vi "Create Plot Object.vi"(6 "Control Ref Queue":T1, 7 "Actual Transform In":T2, 8 "error in (no error)":errorcluster, 9 "Multiplot Representation In":T4, 10 "3D Stem.lvclass in":refnum<class "3D Stem.lvclass">, 11 "Plot Object In":refnum<vi>) -> (0 "error out":errorcluster, 1 "Multiplot Representation Out":T4, 2 "3D Stem.lvclass out":refnum<class "3D Stem.lvclass">, 3 "Plot Object Out":refnum<vi>, 5 "Actual Transform Out":T2)   [LabVIEW 2020, in "3D Stem.lvclass"]
uses:
  <vilib>/Math Plots/3D Math Plots/3D Stem/3D Stem/3D Stem.lvclass
  <vilib>/Math Plots/3D Math Plots/3D Plot/3D Plot/Typedef/Multiplot Representation.ctl
  <vilib>/Math Plots/3D Math Plots/3D Plot/3D Plot/Typedef/Plot Representation.ctl
  <vilib>/Math Plots/3D Math Plots/3D Plot/3D Plot/Typedef/Range Clusters.ctl
  <vilib>/Math Plots/3D Math Plots/3D Plot/3D Plot/Typedef/Mesh Data.ctl
  <vilib>/Math Plots/3D Math Plots/3D Plot/3D Plot/Typedef/Actual Transform.ctl
  <vilib>/Math Plots/3D Math Plots/3D Plot/Action String/3DMathPlot Ctrl Act Queue.ctl
  <vilib>/Math Plots/3D Math Plots/3D Plot/Action String/3DMathPlot Ctrl Act Cluster.ctl
  <vilib>/Math Plots/3D Math Plots/3D Plot/Action String/3DMathPlot State Class.ctl
  <vilib>/Math Plots/3D Math Plots/3D Stem/3D Stem/3D Stem.lvclass/3D Stem.ctl
  <vilib>/Math Plots/3D Math Plots/3D Plot/3D Plot/3D Plot.lvclass
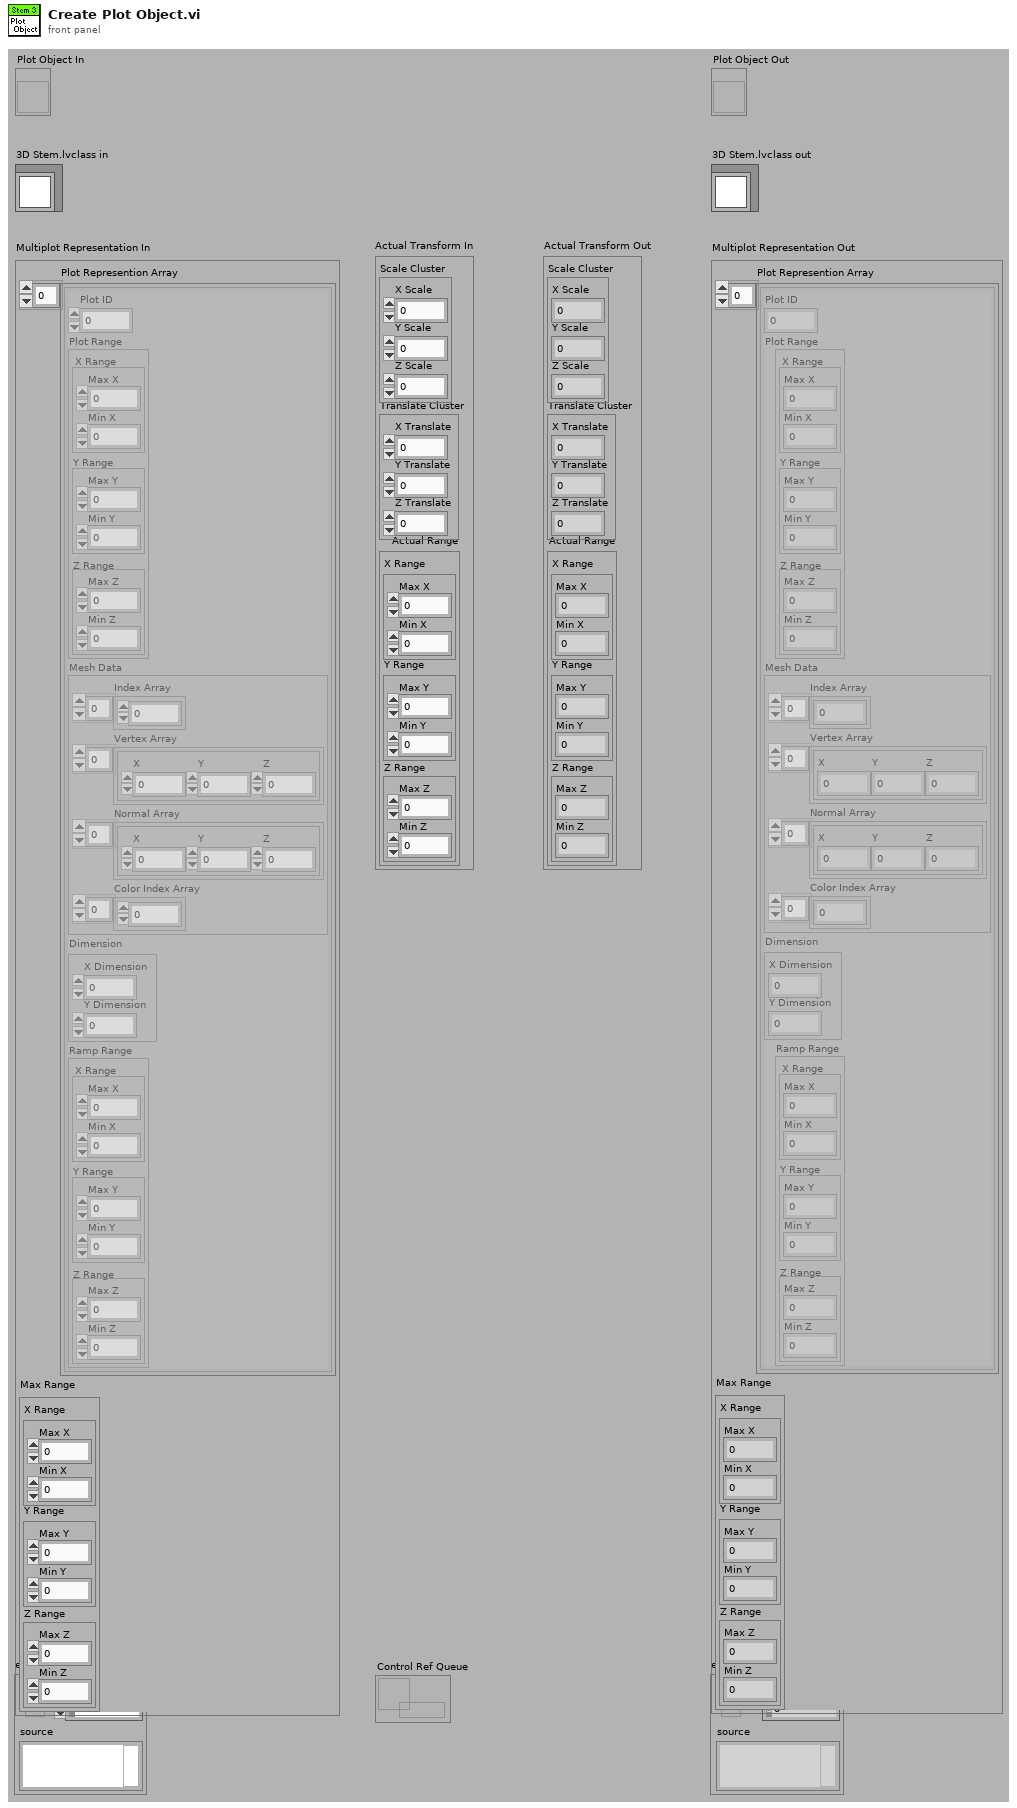
[diagram p1: front panel]
types:
  T1 = typedef "3DMathPlot Ctrl Act Queue.ctl" = refnum<queue>
  T2 = typedef "3D Plot.lvclass/Actual Transform.ctl" = cluster{"Scale Cluster":cluster{"X Scale":sgl, "Y Scale":sgl, "Z Scale":sgl}, "Translate Cluster":cluster{"X Translate":sgl, "Y Translate":sgl, "Z Translate":sgl}, "Actual Range":T3}
  T3 = typedef "3D Plot.lvclass/Range Clusters.ctl" = cluster{"X Range":cluster{"Max X":sgl, "Min X":sgl}, "Y Range":cluster{"Max Y":sgl, "Min Y":sgl}, "Z Range":cluster{"Max Z":sgl, "Min Z":sgl}}
  T4 = typedef "3D Plot.lvclass/Multiplot Representation.ctl" = cluster{"Plot Represention Array":T5[], "Max Range":T3}
  T5 = typedef "3D Plot.lvclass/Plot Representation.ctl" = cluster{"Plot ID":i32, "Plot Range":T3, "Mesh Data":T6, "Dimension":cluster{"X Dimension":i32, "Y Dimension":i32}, "Ramp Range":T3}
  T6 = typedef "3D Plot.lvclass/Mesh Data.ctl" = cluster{"Index Array":u32[], "Vertex Array":cluster{"X":sgl, "Y":sgl, "Z":sgl}[], "Normal Array":cluster{"X":sgl, "Y":sgl, "Z":sgl}[], "Color Index Array":i32[]}
  T7 = typedef "3D Stem.lvclass/3D Stem Property Array.ctl" = T8[]
  T8 = typedef "3D Stem.lvclass/3D Stem Property.ctl" = cluster{"General Property":cluster{"Plot Name":string, "Coordinate System":enum16{"Cartesian", "Cylindrical", "Spherical"}, "Opacity":sgl}, "Projection Property":cluster{"Draw XY":bool, "Draw YZ":bool, "Draw XZ":bool}, "Plot Property":cluster{"Sprite Type":T9, "Point Size":sgl, "Color Ramp Cluster":T10, "Line Style":T11, "Line Width":sgl, "Line Color":u32, "Antialiasing":bool}}
  T9 = typedef "3D Plot.lvclass/Sprite Type.ctl" = enum16{"None", "Empty Square", "Solid Square", "Empty Diamond", "Solid Diamond", "Empty Circle", "Solid Circle", "Asterisk", "Bold X", "Wireframe Sphere", "Solid Sphere", "Wireframe Cube", "Solid Cube"}
  T10 = typedef "3D Plot.lvclass/Color Ramp Cluster.ctl" = cluster{"Color Ramp Style":enum16{"None", "Shaded", "Color spectrum", "Grey scale", "Custom"}, "Color Ramp Array":u32[], "Color Ramp Index":i32[], "Interpolate?":bool, "Logarithm?":bool}
  T11 = typedef "3D Plot.lvclass/Line Type.ctl" = enum16{"None", "Solid", "Dash", "Dot", "Dash Dot"}
  T12 = enum16{"Points", "Lines", "Line Strip", "Line Loop", "Triangles", "Triangle Strip", "Triangle Fan", "Quads", "Quad Strip", "Polygon"}
  T13 = cluster{"Draw XY":bool, "Draw YZ":bool, "Draw XZ":bool}
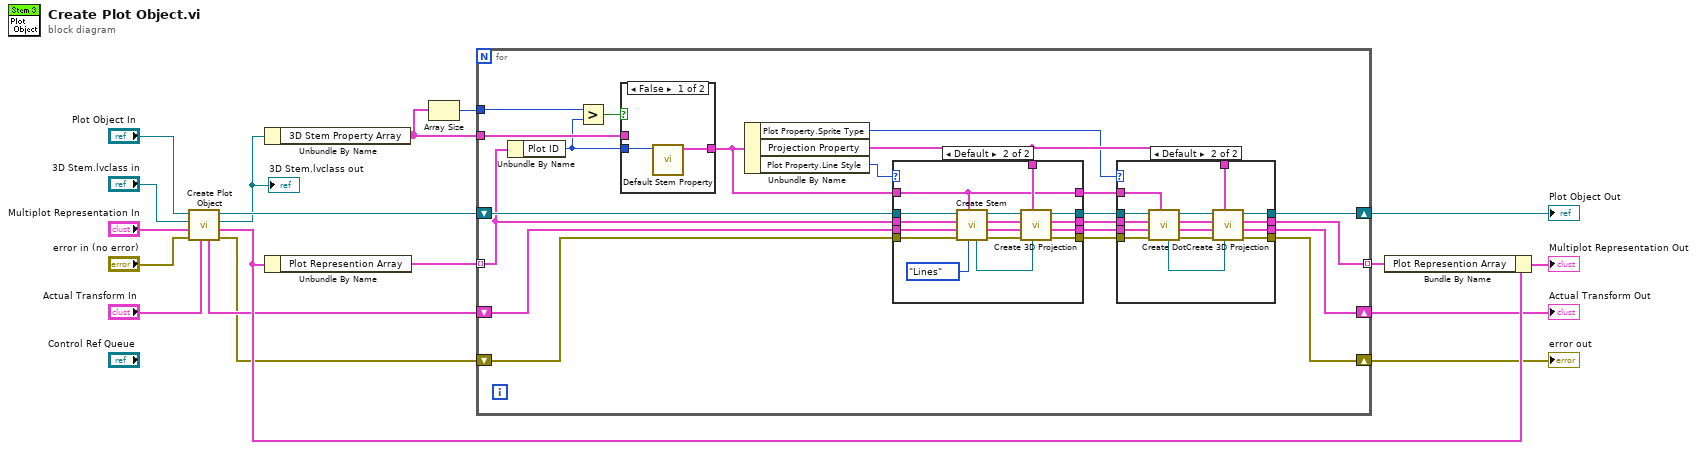
[diagram p0: block diagram]
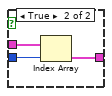
[diagram p2: hidden frame]
diagram:
  n1 = call-parent "Create Plot Object.vi"("Actual Transform In"="Actual Transform In", "error in (no error)"="error in (no error)", "Multiplot Representation In"="Multiplot Representation In", "3D Plot.lvclass in"="3D Stem.lvclass in", "Plot Object In"="Plot Object In") -> ("error out"=w4:errorcluster, "Multiplot Representation Out"=w12:T4, "3D Plot.lvclass out"=w3:refnum<class "3D Stem.lvclass">, "Plot Object Out"=w6:refnum<vi>, "Actual Transform Out"=w9:T2)  [unwired: 2 in]
  "3D Stem.lvclass out" <- w3
  n2 = Unbundle By Name(w3) -> ("3D Stem Property Array"=w2:T7)
  n3 = Unbundle By Name(w12) -> ("Plot Represention Array"=w14:T5[])
  n4 = Array Size(array=w2) -> (size(s)=w1:i32)
  n5 = for {
    shift-right: [w37] -> w7
    shift-left: w4 -> [w33]
    shift-right: [w39] -> w5
    shift-left: w6 -> [w36]
    shift-right: [w38] -> w8
    shift-left: w9 -> [w34]
    tunnel: w14 -> [w35] mode=indexing
    tunnel: w2 -> [w20]
    tunnel: [w31] -> w13 mode=indexing
    tunnel: w1 -> [w21]
    n6 = Unbundle By Name(w35) -> ("Plot ID"=w19:i32)
    n7 = Greater?(x=w21, y=w19) -> (0:w23:bool)
    n8 = case shown="False" w23 {
      tunnel: w20 -> [_ w44]
      tunnel: [w41 w43] -> w22
      tunnel: w19 -> [w40 w42]
      frame False {
        n9 = call <vilib>:"Default Stem Property.vi"("Plot ID"=w40) -> ("Default Property"=w41:T8)  [unwired: 10 out]
      }
      frame True {
        n10 = Index Array(array=w44, index=w42) -> (element=w43:T8)
      }
    }
    n11 = Unbundle By Name(w22) -> ("Plot Property.Sprite Type"=w25:T9, "Projection Property"=w27:T13, "Plot Property.Line Style"=w24:T11)
    n12 = case shown="Default" w24 {
      tunnel: w36 -> [w66 w82]
      tunnel: w35 -> [w65 w81]
      tunnel: w34 -> [w64 w80]
      tunnel: w33 -> [w63 w79]
      tunnel: [w65 w78] -> w32
      tunnel: [w66 w73] -> w30
      tunnel: [w64 w72] -> w29
      tunnel: [w63 w71] -> w28
      tunnel: w27 -> [_ w70]
      tunnel: w22 -> [w67 w68]
      tunnel: [w67 w68] -> w26
      frame "None" {
      }
      frame Default {
        n13 = call <vilib>:"Create Stem.vi"("Draw Mode"=T12."Lines", "3D Stem Property"=w68, "error in (no error)"=w79, "Actual Transform In"=w80, "Plot Representation In"=w81, "Plot Object In"=w82) -> ("error out"=w75:errorcluster, "Actual Transform Out"=w76:T2, "Plot Representation Out"=w78:T5, "Plot Object Out"=w77:refnum<vi>, "Stem Object Out"=w74:refnum<vi>)  [unwired: 1 in]
        n14 = call <vilib>:"Create 3D Projection.vi"("Sub Object In"=w74, "Projection Property"=w70, "error in (no error)"=w75, "Actual Transform In"=w76, "Plot Object In"=w77) -> ("error out"=w71:errorcluster, "Actual Transform Out"=w72:T2, "Plot Object Out"=w73:refnum<vi>)  [unwired: 1 in, 3 out]
      }
    }
    n15 = case shown="Default" w25 {
      tunnel: [w48 w62] -> w39
      tunnel: [w46 w61] -> w38
      tunnel: [w45 w60] -> w37
      tunnel: w32 -> [w47 w59]
      tunnel: [w47 w56] -> w31
      tunnel: w30 -> [w48 w53]
      tunnel: w29 -> [w46 w52]
      tunnel: w28 -> [w45 w51]
      tunnel: w27 -> [_ w50]
      tunnel: w26 -> [_ w49]
      frame "None" {
      }
      frame Default {
        n16 = call <vilib>:"Create Dot.vi"("3D Stem Property"=w49, "error in (no error)"=w51, "Actual Transform In"=w52, "Plot Representation In"=w59, "Plot Object In"=w53) -> ("error out"=w58:errorcluster, "Actual Transform Out"=w57:T2, "Plot Representation Out"=w56:T5, "Plot Object Out"=w55:refnum<vi>, "Dot Object Out"=w54:refnum<vi>)  [unwired: 2 out]
        n17 = call <vilib>:"Create 3D Projection.vi"("Sub Object In"=w54, "Projection Property"=w50, "error in (no error)"=w58, "Actual Transform In"=w57, "Plot Object In"=w55) -> ("error out"=w60:errorcluster, "Actual Transform Out"=w61:T2, "Plot Object Out"=w62:refnum<vi>)  [unwired: 1 in, 3 out]
      }
    }
  }
  "error out" <- w7
  "Plot Object Out" <- w5
  "Actual Transform Out" <- w8
  n18 = Bundle By Name(cluster=w12, "Plot Represention Array"=w13) -> (→"Multiplot Representation Out":T4)
